vi "Merge Errors.vi"(4 "error array in":errorcluster[](array[cluster]) caption="Fehlerarray (Eingang)", 5 "error in 3 (no error)":errorcluster caption="Fehler 3 (Eingang, kein Fehler)", 6 "error in 2 (no error)":errorcluster caption="Fehler 2 (Eingang, kein Fehler)", 7 "error in 1 (no error)":errorcluster caption="Fehler 1 (Eingang, kein Fehler)") -> (0 "error out":errorcluster caption="Fehler (Ausgang)")   [LabVIEW 2009]
doc: "Mit diesem VI können Fehler-I/O-Cluster aus verschiedenen Funktionen zusammengefasst werden."
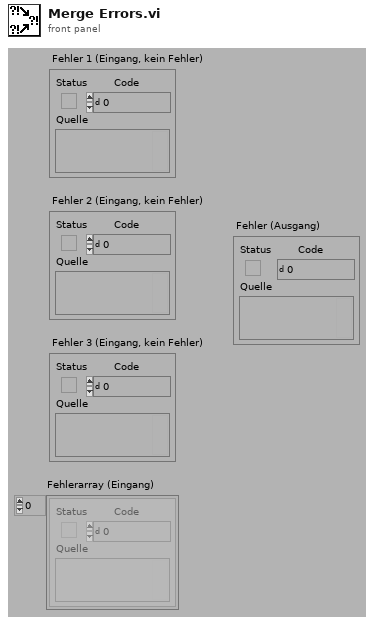
[diagram p1: front panel]
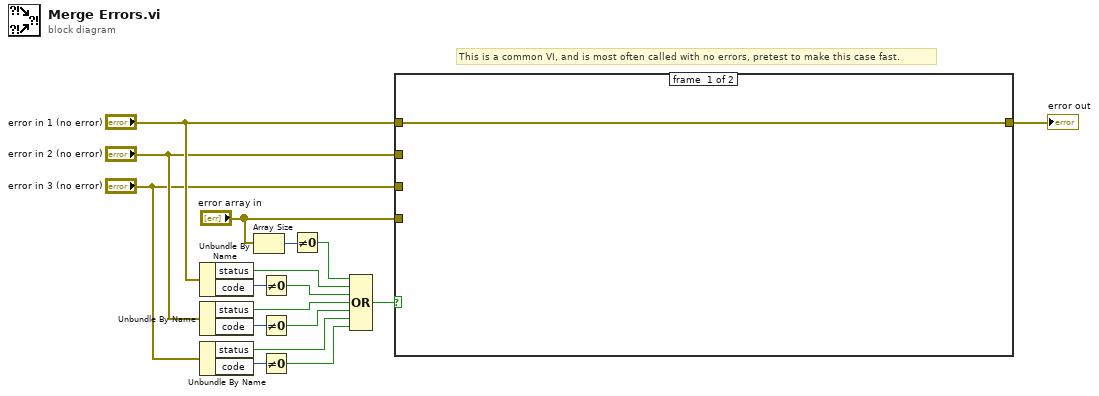
[diagram p0: block diagram]
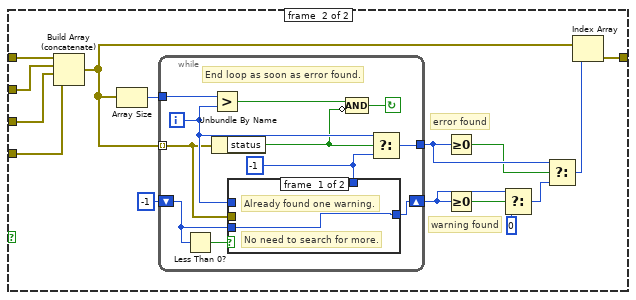
[diagram p2: hidden frame]
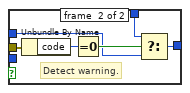
[diagram p3: hidden frame]
diagram:
  # "This is a common VI, and is most often called with no errors, pretest to make this case fast."
  n1 = Unbundle By Name("error in 1 (no error)") -> ("status"=w15:bool, "code"=w8:i32)
  n2 = Unbundle By Name("error in 2 (no error)") -> ("status"=w4:bool, "code"=w7:i32)
  n3 = Unbundle By Name("error in 3 (no error)") -> ("status"=w2:bool, "code"=w6:i32)
  n4 = Array Size(array="error array in") -> (size(s)=w14:i32)
  n5 = Not Equal To 0?(x=w8) -> (x != 0?=w5:bool)
  n6 = Not Equal To 0?(x=w7) -> (x != 0?=w3:bool)
  n7 = Not Equal To 0?(x=w6) -> (x != 0?=w1:bool)
  n8 = Not Equal To 0?(x=w14) -> (x != 0?=w13:bool)
  n9 = Compound Arithmetic op=OR(w13, w15, w5, w4, w3, w2, w1) -> (w12:bool)
  n10 = case shown="True" w12 {
    tunnel: [w18 w33] -> w17
    tunnel: "error in 1 (no error)" -> [w18 w32]
    tunnel: "error in 2 (no error)" -> [_ w31]
    tunnel: "error in 3 (no error)" -> [_ w30]
    tunnel: "error array in" -> [_ w19]
    frame #0 {
    }
    frame #1 {
      # "warning found"
      # "error found"
      n11 = Build Array (concatenate)(w32, w31, w30, w19) -> (w29:errorcluster[])
      n12 = Array Size(array=w29) -> (size(s)=w28:i32)
      n13 = while {
        tunnel: w28 -> [w44]
        tunnel: [w41] -> w27
        tunnel: w29 -> [w37] mode=indexing
        shift-right: [w35] -> w25
        shift-left: -1 -> [w34]
        i -> [w39]
        stop <- w42 continue-if-true
        w40 = -1
        # "End loop as soon as error found."
        n14 = Less Than 0?(x=w34) -> (x < 0?=w36:bool)
        n15 = Greater?(x=w44, y=w39) -> (0:w43:bool)
        n16 = Unbundle By Name(w37) -> ("status"=w38:bool)
        n17 = case shown="True" w36 {
          tunnel: w40 -> [_ w49]
          tunnel: w39 -> [_ w48]
          tunnel: w37 -> [_ w47]
          tunnel: [w45 w46] -> w35
          tunnel: w34 -> [w45 _]
          frame #0 {
            # "No need to search for more."
            # "Already found one warning."
          }
          frame #1 {
            # "Detect warning."
            n18 = Unbundle By Name(w47) -> ("code"=w51:i32)
            n19 = Equal To 0?(x=w51) -> (x = 0?=w50:bool)
            n20 = Select(t=w49, s=w50, f=w48) -> (s? t:f=w46:i32)
          }
        }
        n21 = Compound Arithmetic op=AND(w43, invert w38) -> (w42:bool)
        n22 = Select(t=w39, s=w38, f=w40) -> (s? t:f=w41:i32)
      }
      n23 = Greater Or Equal To 0?(x=w27) -> (x >= 0?=w26:bool)
      n24 = Greater Or Equal To 0?(x=w25) -> (x >= 0?=w24:bool)
      n25 = Select(t=w25, s=w24, f=0) -> (s? t:f=w22:i32)
      n26 = Select(t=w27, s=w26, f=w22) -> (s? t:f=w21:i32)
      n27 = Index Array(array=w29, index=w21) -> (element=w33:errorcluster)
    }
  }
  "error out" <- w17
